vi "Initialise.vi"(8 "error in (no error)":errorcluster, 11 "PWM in":refnum<class "LINX-PCA9865 PWM.lvclass">) -> (0 "error out":errorcluster, 3 "PWM out":refnum<class "LINX-PCA9865 PWM.lvclass">)   [LabVIEW 2019, in "LINX-PCA9865 PWM.lvclass"]
uses:
  LINX-PCA9865 PWM.lvclass
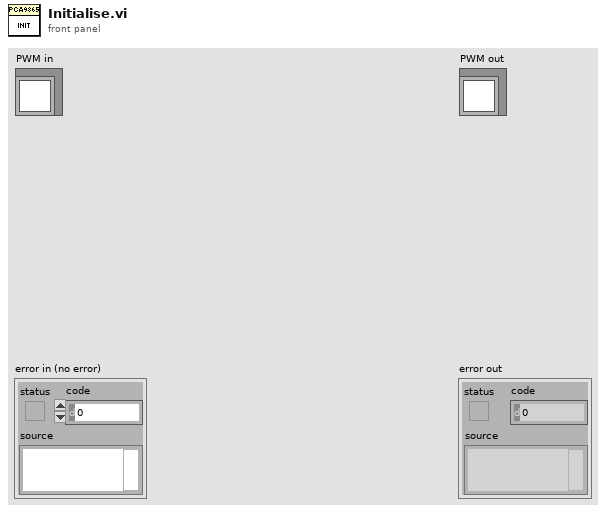
[diagram p1: front panel]
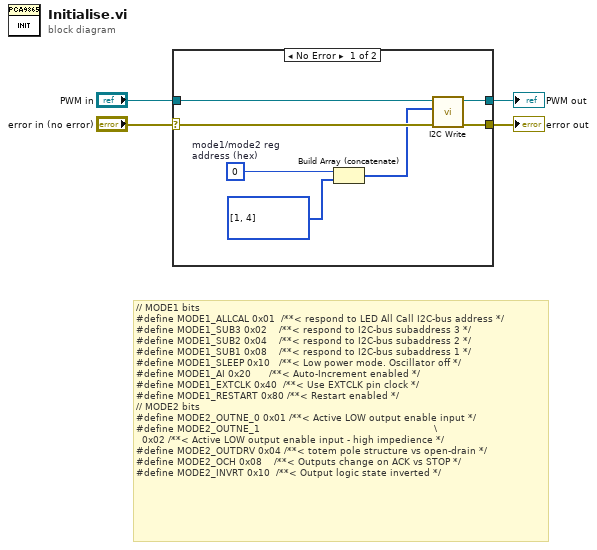
[diagram p0: block diagram]
diagram:
  # "// MODE1 bits\n#define MODE1_ALLCAL 0x01  /**< respond to LED All Call I2C-bus address */\n#define MODE1_SUB3 0x02    /**< respond to I2C-bus subaddress 3 */\n#define MODE1_SUB2 0x04    /**< respond to I2C-bus subaddress 2 */\n#define MODE1_SUB1 0x08    /**< respond to I2C-bus subaddress 1 */\n#define MODE1_SLEEP 0x10   /**< Low power mode. Oscillator off */\n#define MODE1_AI 0x20      /**< Auto-Increment enabled */\n#define MODE1_EXTCLK 0x40  /**< Use EXTCLK pin clock */\n#define MODE1_RESTART 0x80 /**< Restart enabled */\n// MODE2 bits\n#define MODE2_OUTNE_0 0x01 /**< Active LOW output enable input */\n#define MODE2_OUTNE_1                                                          \\\n  0x02 /**< Active LOW output enable input - high impedience */\n#define MODE2_OUTDRV 0x04 /**< totem pole structure vs open-drain */\n#define MODE2_OCH 0x08    /**< Outputs change on ACK vs STOP */\n#define MODE2_INVRT 0x10  /**< Output logic state inverted */"
  n1 = case shown="No Error" "error in (no error)" {
    selector: "error in (no error)" -> [w10 w13]
    tunnel: [w9 w13] -> w3
    tunnel: [w8 w12] -> w1
    tunnel: "PWM in" -> [w11 w12]
    frame No Error {
      w6 = u8 0  # mode1/mode2 reg address (hex)
      n2 = Build Array (concatenate)(w6, u8[] [1, 4] ("Data")) -> (w5:u8[])
      n3 = call "I2C Write.vi"("error in (no error)"=w10, "Bytes to Write"=w5, "LINX-PCA9865 PWM in"=w11) -> ("error out"=w9:errorcluster, "LINX-PCA9865 PWM out"=w8:refnum<class "LINX-PCA9865 PWM.lvclass">)  [unwired: 7 in]
    }
    frame Error {
    }
  }
  "error out" <- w3
  "PWM out" <- w1
